vi "GDSLvLib_ReadLibType.vi"(0 "Class Refnum In":refnum<vi>, 5 "error in (no error)":errorcluster) -> (14 "Class Refnum Out":refnum<vi>, 15 "LibSettings":T1, 19 "error out":errorcluster)   [LabVIEW 2014]
uses:
  <resource>/Framework/Providers/Open_GDS/ClassProviders/Common/LvLib_class/GDSLvLib_LibSettingsType.ctl
  <resource>/Framework/Providers/Open_GDS/ClassProviders/Common/LvClass_class/GDSLvClass_PlugIn.ctl
  <resource>/Framework/Providers/Open_GDS/ClassProviders/Common/LvClass_class/GDSLvClass_PlugInTypes.ctl
  <resource>/Framework/Providers/Open_GDS/ClassProviders/Common/LvLib_class/GDSLvLib_LibTypeSettingNames.ctl
  <resource>/Framework/Providers/Open_GDS/ClassProviders/Provider_LvNativeClass/LvNativeProviderName.ctl
  <resource>/Framework/Providers/Open_GDS/ClassProviders/Common/ScriptingFunctions/Scripting_ConnectorPanePatternType.ctl
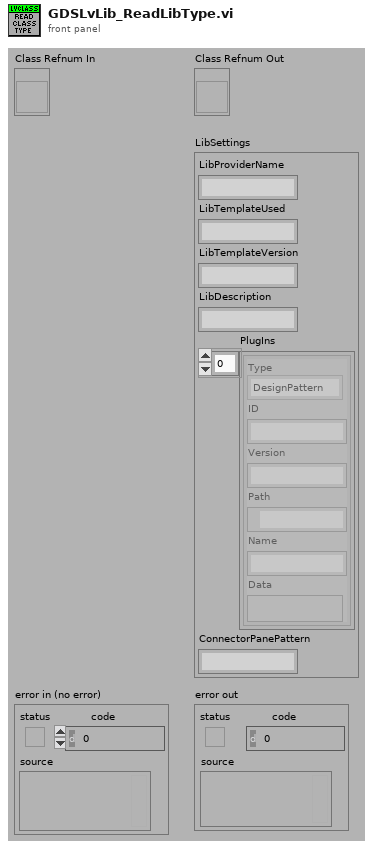
[diagram p1: front panel]
types:
  T1 = typedef "GDSLvLib_LibSettingsType.ctl" = cluster{"LibProviderName":string, "LibTemplateUsed":string, "LibTemplateVersion":string, "LibDescription":string, "PlugIns":T2[], "ConnectorPanePattern":string}
  T2 = typedef "GDSLvClass_PlugIn.ctl" = cluster{"Type":T3, "ID":string, "Version":string, "Path":path, "Name":string, "Data":variant}
  T3 = typedef "GDSLvClass_PlugInTypes.ctl" = enum16{"DesignPattern", "MethodTypes"}
  T4 = typedef "GDSLvLib_LibTypeSettingNames.ctl" = enum16{"EndevoGOOP_LibProvider", "EndevoGOOP_TemplateUsed", "EndevoGOOP_TemplateVersion", "EndevoGOOP_PlugIns", "EndevoGOOP_ConnectorPanePattern"}
  T5 = typedef "LvNativeProviderName.ctl" = enum16{"Endevo LabVIEW Native"}
  T6 = typedef "Scripting_ConnectorPanePatternType.ctl" = u16
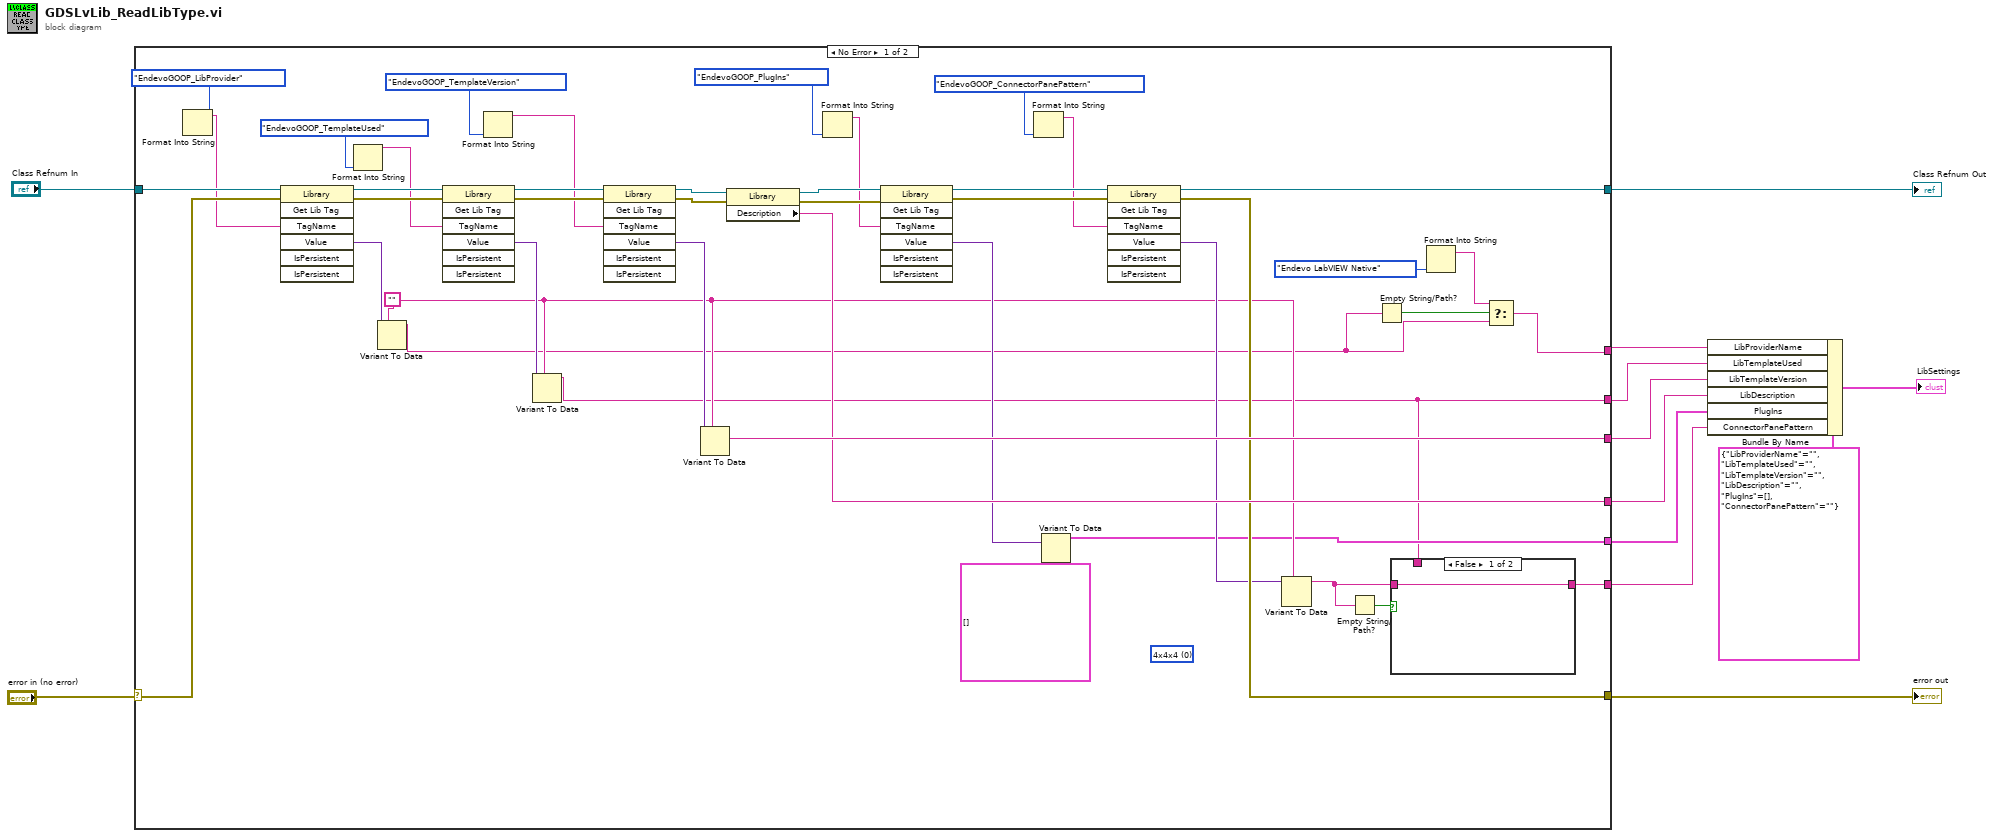
[diagram p0: block diagram]
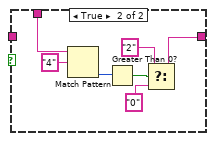
[diagram p2: hidden frame]
diagram:
  n1 = case shown="No Error" "error in (no error)" {
    selector: "error in (no error)" -> [w55 w65]
    tunnel: [w31 w65] -> w11
    tunnel: "Class Refnum In" -> [w50 w64]
    tunnel: [w30 w64] -> w9
    tunnel: [w18 _] -> w8
    tunnel: [w47 _] -> w7
    tunnel: [w21 _] -> w3
    tunnel: [w44 _] -> w6
    tunnel: [w26 _] -> w5
    tunnel: [w22 _] -> w4
    frame No Error {
      (unwired) T6 0 items=["4x4x4", "5x6x5", "6x8x6"] ("Pattern")
      w27 = ""
      n2 = Format Into String(GDSLvLib_LibTypeSettingNames."EndevoGOOP_LibProvider" ("ClassTypeSettingNames")) -> (resulting string=w40:string)  [unwired: 3 in, 1 out]
      n3 = invoke class="Library" method="Get Lib Tag"(reference=w50, error in=w55, "TagName"=w40) -> (reference out=w54:refnum<vi>, error out=w53:errorcluster, "Value"=w52:variant)  [unwired: 4 in, 4 out]
      n4 = Format Into String(GDSLvLib_LibTypeSettingNames."EndevoGOOP_TemplateUsed" ("ClassTypeSettingNames")) -> (resulting string=w38:string)  [unwired: 3 in, 1 out]
      n5 = Variant To Data(type=w27, Variant=w52) -> (data=w19:string)  [unwired: 1 in, 1 out]
      n6 = invoke class="Library" method="Get Lib Tag"(reference=w54, error in=w53, "TagName"=w38) -> (reference out=w49:refnum<vi>, error out=w48:errorcluster, "Value"=w51:variant)  [unwired: 4 in, 4 out]
      n7 = Format Into String(GDSLvLib_LibTypeSettingNames."EndevoGOOP_TemplateVersion" ("ClassTypeSettingNames")) -> (resulting string=w39:string)  [unwired: 3 in, 1 out]
      n8 = Variant To Data(type=w27, Variant=w51) -> (data=w21:string)  [unwired: 1 in, 1 out]
      n9 = invoke class="Library" method="Get Lib Tag"(reference=w49, error in=w48, "TagName"=w39) -> (reference out=w46:refnum<vi>, error out=w45:errorcluster, "Value"=w43:variant)  [unwired: 4 in, 4 out]
      n10 = Variant To Data(type=w27, Variant=w43) -> (data=w47:string)  [unwired: 1 in, 1 out]
      n11 = property class="Library"(reference=w46, error in=w45) -> (reference out=w37:refnum<vi>, error out=w36:errorcluster, "Description"=w44:string)
      n12 = Format Into String(GDSLvLib_LibTypeSettingNames."EndevoGOOP_PlugIns" ("ClassTypeSettingNames")) -> (resulting string=w35:string)  [unwired: 3 in, 1 out]
      n13 = invoke class="Library" method="Get Lib Tag"(reference=w37, error in=w36, "TagName"=w35) -> (reference out=w33:refnum<vi>, error out=w32:errorcluster, "Value"=w34:variant)  [unwired: 4 in, 4 out]
      n14 = Format Into String(GDSLvLib_LibTypeSettingNames."EndevoGOOP_ConnectorPanePattern" ("ClassTypeSettingNames")) -> (resulting string=w29:string)  [unwired: 3 in, 1 out]
      n15 = Variant To Data(type=T2[] [] ("PlugIns"), Variant=w34) -> (data=w26:T2[])  [unwired: 1 in, 1 out]
      n16 = invoke class="Library" method="Get Lib Tag"(reference=w33, error in=w32, "TagName"=w29) -> (reference out=w30:refnum<vi>, error out=w31:errorcluster, "Value"=w28:variant)  [unwired: 4 in, 4 out]
      n17 = Variant To Data(type=w27, Variant=w28) -> (data=w23:string)  [unwired: 1 in, 1 out]
      n18 = Empty String/Path?(string/path=w23) -> (empty?=w24:bool)
      n19 = Empty String/Path?(string/path=w19) -> (empty?=w20:bool)
      n20 = case shown="False" w24 {
        tunnel: w23 -> [w56 _]
        tunnel: [w56 w59] -> w22
        tunnel: w21 -> [_ w63]
        frame False {
        }
        frame True {
          n21 = Match Pattern(string=w63, regular expression="4") -> (offset past match=w61:i32)  [unwired: 1 in, 3 out]
          n22 = Greater Than 0?(x=w61) -> (x > 0?=w60:bool)
          n23 = Select(t="2", s=w60, f="0" ("regular expression")) -> (s? t:f=w59:string)
        }
      }
      n24 = Format Into String(LvNativeProviderName."Endevo LabVIEW Native" ("ProviderName")) -> (resulting string=w16:string)  [unwired: 3 in, 1 out]
      n25 = Select(t=w16, s=w20, f=w19) -> (s? t:f=w18:string)
    }
    frame Error {
    }
  }
  "Class Refnum Out" <- w9
  "error out" <- w11
  n26 = Bundle By Name(cluster=T1 {"LibProviderName"="", "LibTemplateUsed"="", "LibTemplateVersion"="", "LibDescription"="", "PlugIns"=[], "ConnectorPanePattern"=""} ("LibSettings"), "LibProviderName"=w8, "LibTemplateUsed"=w3, "LibTemplateVersion"=w7, "LibDescription"=w6, "PlugIns"=w5, "ConnectorPanePattern"=w4) -> (→"LibSettings":T1)
